vi "NewTimer.vi"() -> ()   [LabVIEW 2011]
panel:
  out "Time":timestamp
  out "range element(true=In Range)":bool[](array[boolean])
  out "any one In Range?( true=In Range)":bool
  out "any overlay? (true=no overlay)":bool
  out "overlay element(true=no overlay)":bool[](array[boolean])
  in  "stop":bool
  out "Array 2":timestamp[](array[timestamp])
  in  "Array":timestamp[][](array[timestamp]) format="%<%I:%M %p>T"
  # "srart"
  # "end"
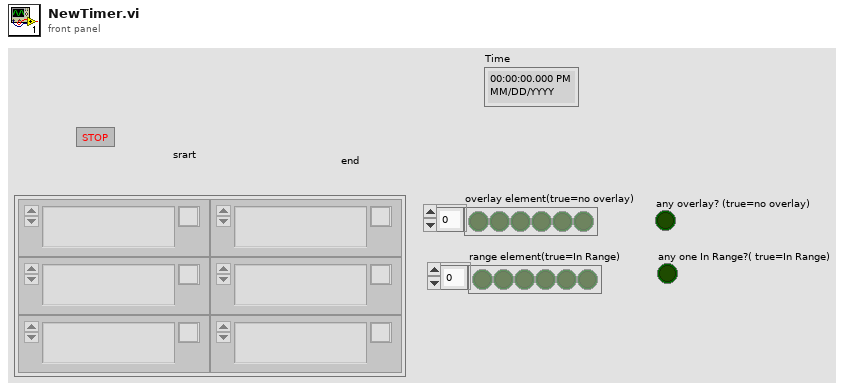
[diagram p1: front panel]
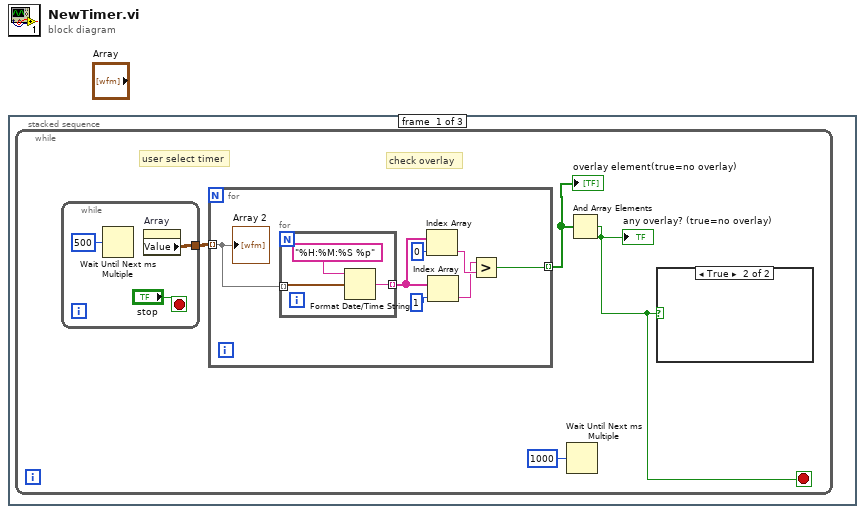
[diagram p0: block diagram]
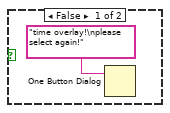
[diagram p2: hidden frame]
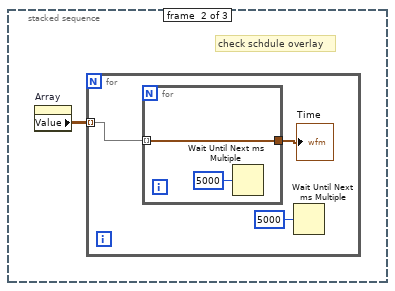
[diagram p3: hidden frame]
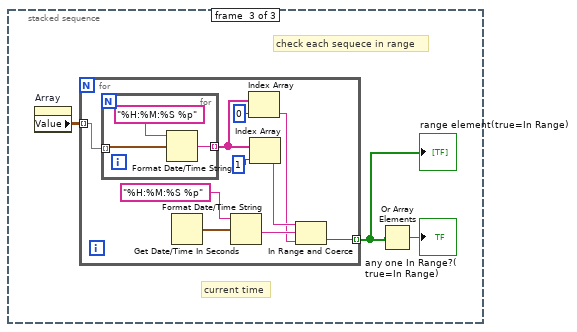
[diagram p4: hidden frame]
diagram:
  n1 = stacked-sequence {
    frame #0 {
      n2 = while {
        stop <- w1 stop-if-true
        # "user select timer"
        # "check overlay"
        n3 = while {
          tunnel: [w6] -> w4
          stop <- "stop" stop-if-true
          n4 = Wait Until Next ms Multiple(millisecond multiple=u32 500 ("millisecond timer value")) -> ()  [unwired: 1 out]
          n5 = property on="Array" class="Arr (strict)"() -> ("Value"=w6:timestamp[][])  [unwired: 2 in, 2 out]
        }
        n6 = for {
          tunnel: w4 -> [w15] mode=indexing
          tunnel: [w11] -> w3 mode=indexing
          n7 = for {
            tunnel: w15 -> [w18] mode=indexing
            tunnel: [w16] -> w13 mode=indexing
            n8 = Format Date/Time String(time format string (%c)="%H:%M:%S %p", seconds (now)=w18) -> (date/time string=w16:string)  [unwired: 1 in]
          }
          n9 = Index Array(array=w13, index=0) -> (element=w10:string)
          n10 = Index Array(array=w13, index=1) -> (element=w9:string)
          n11 = Greater?(x=w9, y=w10) -> (0:w11:bool)
          "Array 2" <- w15
        }
        "overlay element(true=no overlay)" <- w3
        n12 = Wait Until Next ms Multiple(millisecond multiple=u32 1000) -> ()  [unwired: 1 out]
        n13 = And Array Elements(Boolean array=w3) -> (logical AND=w1:bool)
        "any overlay? (true=no overlay)" <- w1
        n14 = case shown="True" w1 {
          frame False {
            n15 = One Button Dialog(message="time overlay!\nplease select again!") -> ()  [unwired: 1 in, 1 out]
          }
          frame True {
          }
        }
      }
    }
    frame #1 {
      # "check schdule overlay"
      n16 = property on="Array" class="Arr (strict)"() -> ("Value"=w19:timestamp[][])  [unwired: 2 in, 2 out]
      n17 = for {
        tunnel: w19 -> [w22] mode=indexing
        n18 = for {
          tunnel: w22 -> [w23] mode=indexing
          tunnel: [w23] -> w21
          n19 = Wait Until Next ms Multiple(millisecond multiple=u32 5000) -> ()  [unwired: 1 out]
        }
        "Time" <- w21
        n20 = Wait Until Next ms Multiple(millisecond multiple=u32 5000) -> ()  [unwired: 1 out]
      }
    }
    frame #2 {
      # "current time"
      # "check each sequece in range"
      n21 = property on="Array" class="Arr (strict)"() -> ("Value"=w27:timestamp[][])  [unwired: 2 in, 2 out]
      n22 = for {
        tunnel: w27 -> [w34] mode=indexing
        tunnel: [w29] -> w26 mode=indexing
        n23 = for {
          tunnel: w34 -> [w40] mode=indexing
          tunnel: [w38] -> w36 mode=indexing
          n24 = Format Date/Time String(time format string (%c)="%H:%M:%S %p", seconds (now)=w40) -> (date/time string=w38:string)  [unwired: 1 in]
        }
        n25 = Get Date/Time In Seconds() -> (seconds since 1Jan1904=w28:timestamp)
        n26 = Format Date/Time String(time format string (%c)="%H:%M:%S %p", seconds (now)=w28) -> (date/time string=w32:string)  [unwired: 1 in]
        n27 = Index Array(array=w36, index=0) -> (element=w30:string)
        n28 = Index Array(array=w36, index=1) -> (element=w31:string)
        n29 = In Range and Coerce(upper limit=w31, x=w32, lower limit=w30) -> (In Range?=w29:bool)  [unwired: 1 out]
      }
      "range element(true=In Range)" <- w26
      n30 = Or Array Elements(Boolean array=w26) -> (logical OR=→"any one In Range?( true=In Range)":bool)
    }
  }
